vi "savebinaryfiles.vi"   [LabVIEW 2015]
types:
  T1 = typedef "LVRectTypeDef.ctl" = cluster{"Left":i16, "Top":i16, "Right":i16, "Bottom":i16}
  T2 = cluster{"Xpixels":i32, "Vxminref":dbl, "Vxmaxref":dbl, "P":dbl, "Ypixels":i32, "Vyminref":dbl, "Vymaxref":dbl, "srate":sgl, "sAOxy":i32, "timeout":dbl, "type":string, "date":string, "time":string, "Colormap":u16, "Drawing Mode":u16, "Scanning Mode":u16, "square pixels":bool, "square matrix":bool, "Xpixels Img":i32, "Vx-min Img":dbl, "VX-max Img":dbl, "Ypixels Img":i32, "Vy-min Img":dbl, "Vy-max Img ":dbl, "Angle Img":dbl, "autoshutter":bool, "finite":bool, "cont":bool, "wavdet":bool, "measpoints":i32, "avpp":i32, "bufferAO":i32, "bufferAI":i32, "starttick":u32, "waveform":path, "Vx-ref":dbl, "Vy-ref":dbl, "refreshrate":dbl, "refreshbuffer":i32, "tt_cycles":i32, "motorref":refnum<k7>, "mirrorswitch":refnum<k7>, "sample mode":i32, "maxbufferAI":i32, "srateAODO":sgl, "bin":sgl, "Pel":sgl, "Angle draw":dbl, "srate Img":sgl, "ROIimg_plotbounds":T1, "auto OD":bool, "ODfilt":u16, "aAI":i32[], "aCI":i32[], "aAO":u32[], "aDO":u32[], "refwfsize":dbl, "Lifetime":bool, "Vz-Img":dbl, "Vz-ref":dbl, "Vz-reset":dbl, "AIoverride":bool, "aAS":u32[], "XYZstart":dbl[], "External 100KHz Clock?":bool}
  T3 = cluster{"E_binfile":errorcluster[], "binfile":refnum<file>[]}
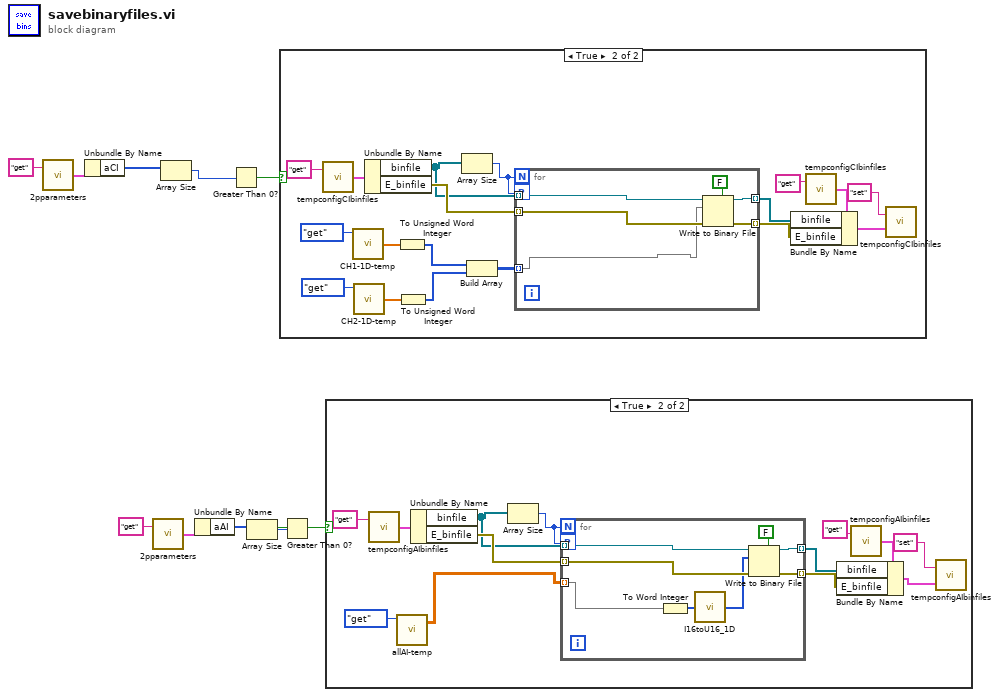
[diagram p0: block diagram]
diagram:
  n1 = call "2pparameters.vi"("command"="get") -> ("params out"=w4:T2)  [unwired: 1 in]
  n2 = Unbundle By Name(w4) -> ("aCI"=w5:i32[])
  n3 = call "2pparameters.vi"("command"="get") -> ("params out"=w9:T2)  [unwired: 1 in]
  n4 = Array Size(array=w5) -> (size(s)=w2:i32)
  n5 = Unbundle By Name(w9) -> ("aAI"=w8:i32[])
  n6 = Greater Than 0?(x=w2) -> (x > 0?=w1:bool)
  n7 = Array Size(array=w8) -> (size(s)=w7:i32)
  n8 = case shown="True" w1 {
    frame False {
    }
    frame True {
      n9 = call "tempconfigCIbinfiles.vi"("command"="get") -> ("Temp Config out"=w27:T3)  [unwired: 1 in]
      n10 = call "CH1-1D-temp.vi"("command"=enum16{"get", "set", "clear", "append"}."get") -> ("array out"=w14:sgl[])  [unwired: 3 in, 1 out]
      n11 = call "CH2-1D-temp.vi"("command"=enum16{"get", "set", "clear", "append"}."get") -> ("array out"=w15:sgl[])  [unwired: 3 in, 1 out]
      n12 = Unbundle By Name(w27) -> ("binfile"=w23:refnum<file>[], "E_binfile"=w28:errorcluster[])
      n13 = To Unsigned Word Integer(number=w14) -> (unsigned 16bit integer=w16:u16[])
      n14 = To Unsigned Word Integer(number=w15) -> (unsigned 16bit integer=w17:u16[])
      n15 = Array Size(array=w23) -> (size(s)=w22:i32)
      n16 = Build Array(w16, w17) -> (w13:u16[][])
      n17 = for {
        N: w22 -> [_]
        tunnel: w28 -> [w34] mode=indexing
        tunnel: w23 -> [w33] mode=indexing
        tunnel: [w31] -> w25 mode=indexing
        tunnel: [w30] -> w24 mode=indexing
        workers-P: w22 -> [_]
        tunnel: w13 -> [w29] mode=indexing
        n18 = Write to Binary File(file (use dialog)=w33, data=w29, error in=w34, 5:FALSE ("prepend array or string size? (T)")) -> (refnum out=w31:refnum<file>, error out=w30:errorcluster)  [unwired: 2 in, 1 out]
      }
      n19 = call "tempconfigCIbinfiles.vi"("command"="get") -> ("Temp Config out"=w19:T3)  [unwired: 1 in]
      n20 = Bundle By Name(cluster=w19, "binfile"=w25, "E_binfile"=w24) -> (w21:T3)
      n21 = call "tempconfigCIbinfiles.vi"("Temp Config in"=w21, "command"="set") -> ()  [unwired: 1 out]
    }
  }
  n22 = Greater Than 0?(x=w7) -> (x > 0?=w6:bool)
  n23 = case shown="True" w6 {
    frame False {
    }
    frame True {
      n24 = call "tempconfigAIbinfiles.vi"("command"="get") -> ("Temp Config out"=w46:T3)  [unwired: 1 in]
      n25 = call "allAI-temp.vi"("command"=enum16{"get", "set", "clear", "append"}."get") -> ("array out"=w35:sgl[][])  [unwired: 3 in, 1 out]
      n26 = Unbundle By Name(w46) -> ("binfile"=w38:refnum<file>[], "E_binfile"=w47:errorcluster[])
      n27 = Array Size(array=w38) -> (size(s)=w37:i32)
      n28 = for {
        N: w37 -> [_]
        tunnel: w47 -> [w55] mode=indexing
        tunnel: w38 -> [w54] mode=indexing
        tunnel: [w52] -> w42 mode=indexing
        tunnel: [w51] -> w41 mode=indexing
        tunnel: w35 -> [w50] mode=indexing
        workers-P: w37 -> [_]
        n29 = To Word Integer(number=w50) -> (16bit integer=w49:i16[])
        n30 = call "I16toU16_1D.vi"("I16"=w49) -> ("U16"=w48:u16[])
        n31 = Write to Binary File(file (use dialog)=w54, data=w48, error in=w55, 5:FALSE ("prepend array or string size? (T)")) -> (refnum out=w52:refnum<file>, error out=w51:errorcluster)  [unwired: 2 in, 1 out]
      }
      n32 = call "tempconfigAIbinfiles.vi"("command"="get") -> ("Temp Config out"=w43:T3)  [unwired: 1 in]
      n33 = Bundle By Name(cluster=w43, "binfile"=w42, "E_binfile"=w41) -> (w39:T3)
      n34 = call "tempconfigAIbinfiles.vi"("Temp Config in"=w39, "command"="set") -> ()  [unwired: 1 out]
    }
  }
